vi "PSK_Mod_Receive_queue.vi"() -> ()   [LabVIEW 2014]
uses:
  <vilib>/addons/Modulation/Digital/General/MT Generate Bits (Galois, PN Order).vi
  <vilib>/addons/Modulation/Digital/Support/Common/Validators/mod_Generate Bits Validate.vi
  <vilib>/addons/Modulation/Analog/support/mod_Set Error Source.vi
  <vilib>/addons/Modulation/Digital/General/MT Generate PSK System Parameters(M).vi
  <vilib>/addons/Modulation/Digital/Support/Common/Validators/mod_Generate Filter Coefficients Validate.vi
  <vilib>/addons/Modulation/Digital/General/subVIs/mod_Generate Filter Coefficients.vi
  <vilib>/addons/Modulation/Digital/General/subVIs/mod_Generate Bits PN Sequence.vi
  <vilib>/addons/Modulation/Digital/General/MT Generate PSK Synchronization Parameters (bit array).vi
  <instrlib>/niUSRP/niUSRP Fetch Rx Data (CDB Cluster).vi
  <vilib>/addons/Modulation/niDMT.lvlib
  <vilib>/addons/Modulation/niAMT.lvlib
panel:
  out "Demod loop time":dbl
  out "USRP loop time":dbl
  out "Lost packets":u32
  in  "Header bits":i32=16
  in  "stop":bool
  out "Packets received":i32
  out "bits received":i32
  out "Aquisition time":dbl
  out "Array":i8[][](array[numeric])
  in  "Message bits":i32=128
  in  "Sync bits":i32=30
  out "sync correct?":bool
  out "output bit stream":i8[](array[numeric])
  out "Before demod&compensation":waveform(dbl)(graph)
  out "Constellation Graph":T1(graph) caption="Rx Signal Constellation"
  out "error out":errorcluster={"status"=FALSE, "code"=1074118647, "source"="niUSRP Fetch Rx Data (CDB Cluster).vi<ERR>Overflow: an internal receive buffer has filled before the data could be returned.  Consider reducing the IQ rate, increasing the Fetch rate, or increasing the number of samples per Fetch."}
  in  "USRP IP Address":refnum<k15>="192.168.10.1"
  out "Actual Rx Parameters":T2={"Rx IQ Sampling\nRate [s/sec]"=200000.0, "Rx\nFrequency [Hz]"=915000000.0, "Rx Gain [dB]"=20.0, "Rx Antenna"="RX1"} {"Rx Gain [dB]" format="%#.6p"; "Rx\nFrequency [Hz]" format="%#.6p"; "Rx IQ Sampling\nRate [s/sec]" format="%#.6p"}
  in  "Rx Parameters":T2={"Rx IQ Sampling\nRate [s/sec]"=400000.0, "Rx\nFrequency [Hz]"=5795000000.0, "Rx Gain [dB]"=0.0, "Rx Antenna"="RX1"} {"Rx Gain [dB]" format="%#.6p"; "Rx\nFrequency [Hz]" format="%#.6p"; "Rx IQ Sampling\nRate [s/sec]" format="%#.6p"}
  in  "Packets per burst":i32=20
  in  "filter parameters":T3={"Alpha"=0.5, "Filter Length"=6, "TX Filter"=enum."Root Raised Cos"} {"Alpha" format="%.2f"}
  in  "QPSK System Parameters":T4={"Samples per Symbol"=8, "symbol map"=[], "Differential PSK"=enum."disable", "PSK type"=0} {"PSK type" items=["normal", "shifted", "offset"]; "symbol map" format="%.3f"}
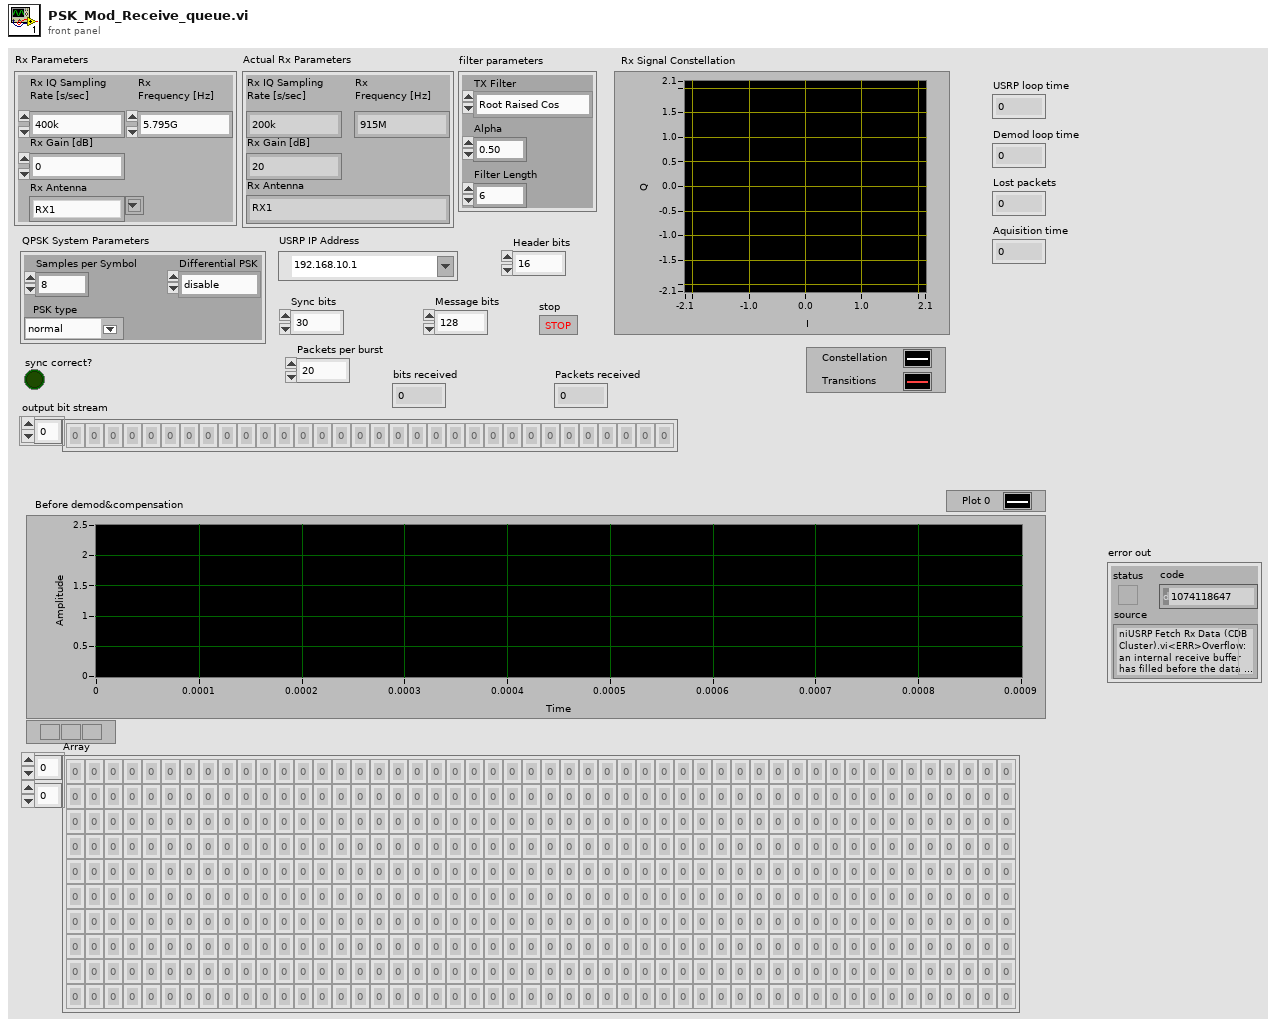
[diagram p1: front panel]
types:
  T1 = cluster{"constellation":dbl[], "oversampled data":dbl[]}[]
  T2 = cluster{"Rx IQ Sampling\nRate [s/sec]":dbl, "Rx\nFrequency [Hz]":dbl, "Rx Gain [dB]":dbl, "Rx Antenna":string}
  T3 = cluster{"Alpha":dbl, "Filter Length":i32, "TX Filter":enum16{"none", "Raised Cosine", "Root Raised Cos", "Gaussian"}}
  T4 = cluster{"Samples per Symbol":i32, "symbol map":cdb[], "Differential PSK":enum16{"disable", "enable"}, "PSK type":u16}
  T5 = enum16{"FSK", "PSK", "QAM", "MSK", "PAM", "ASK", "CPM"}
  T6 = enum16{"none", "Raised Cosine", "Root Raised Cos", "Gaussian"}
  T7 = cluster{"samples per symbol (16)":i32, "symbol map":cdb[], "differential PSK":enum16{"disable", "enable"}, "PSK type":u16}
  T8 = cluster{"expected sync location (symbols)":i32, "sync sequence":cdb[], "sync location uncertainty (symbols)":i32, "sync indent (symbols)":i32}
  T9 = typedef "niAMT.lvlib/Complex Data Waveform.ctl" = cluster{"t0":dbl, "dt":dbl, "Y":cdb[]}
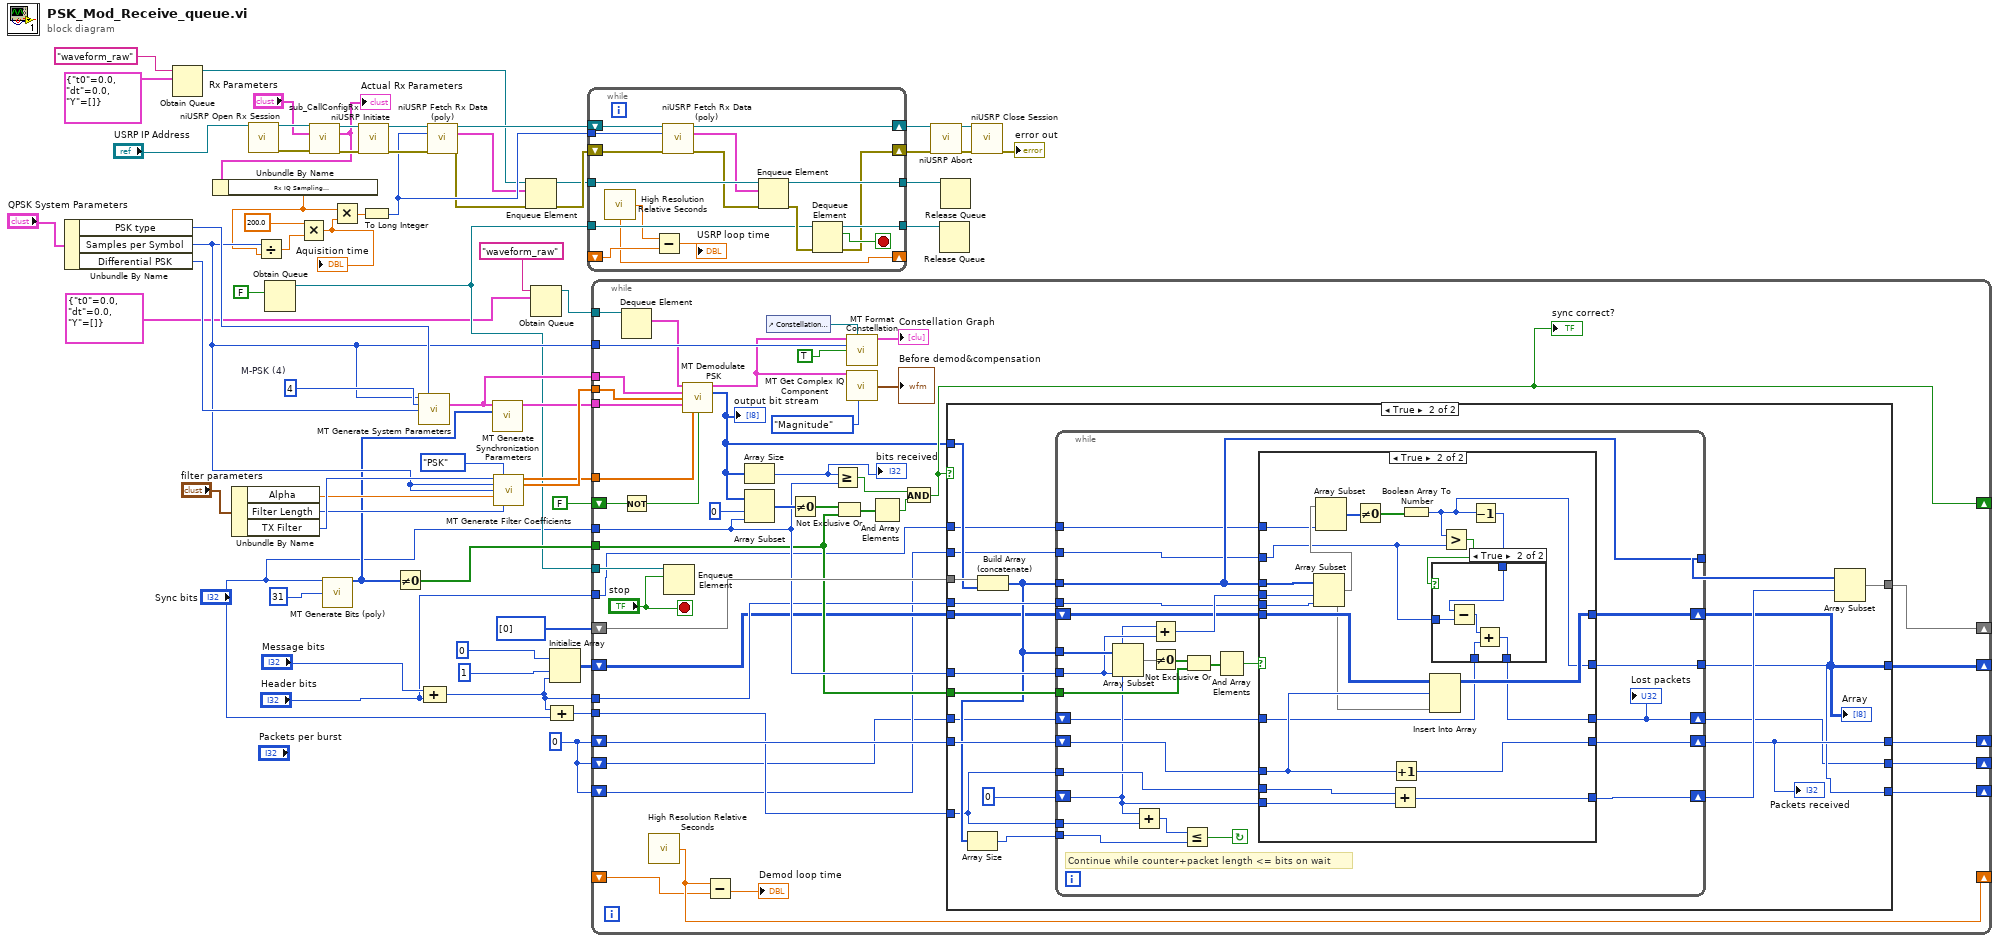
[diagram p0: block diagram]
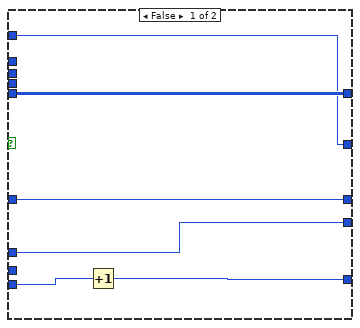
[diagram p3: hidden frame]
diagram:
  w5 = 0
  w61 = 4  # M-PSK (4)
  n1 = Unbundle By Name("QPSK System Parameters") -> ("PSK type"=w36:u16, "Samples per Symbol"=w33:i32, "Differential PSK"=w62:enum16{"disable", "enable"})
  n2 = Obtain Queue(name (unnamed)="waveform_raw", element data type=cluster{"t0":dbl, "dt":dbl, "Y":cdb[]} {"t0"=0.0, "dt"=0.0, "Y"=[]} ("data")) -> (queue out=w25:refnum<queue>)  [unwired: 3 in, 2 out]
  n3 = Unbundle By Name("filter parameters") -> ("Alpha"=w58:dbl, "Filter Length"=w59:i32, "TX Filter"=w60:T6)
  n4 = call <instrlib>:"niUSRP Open Rx Session.vi"("device names"="USRP IP Address") -> ("session handle out"=w52:refnum<k15>, "error out"=w53:errorcluster)  [unwired: 13 in]
  n5 = Obtain Queue(element data type=FALSE) -> (queue out=w12:refnum<queue>)  [unwired: 4 in, 2 out]
  n6 = call "sub_CallConfigRx.vi"("session handle"=w52, "Rx Parameters"="Rx Parameters", "error in"=w53) -> ("session handle out"=w50:refnum<k15>, "Actual Rx Parameters"=w47:T2, "error out"=w49:errorcluster)  [unwired: 10 in]
  "Actual Rx Parameters" <- w47
  n7 = Unbundle By Name(w47) -> ("Rx IQ Sampling\nRate [s/sec]"=w20:dbl)
  n8 = Divide(x=w33, y=w20) -> (x/y=w31:dbl)
  n9 = Multiply(x=200.0, y=w31) -> (x*y=w4:dbl)
  "Aquisition time" <- w4
  n10 = call-poly <vilib>:"MT Generate Bits (poly).vi"("total bits (128)"="Sync bits", "PN sequence order (9)"=31) -> ("output bit stream"=w14:i8[])  [unwired: 11 in, 2 out]
  n11 = Multiply(x=w20, y=w4) -> (x*y=w54:dbl)
  n12 = call <instrlib>:"niUSRP Initiate.vi"("session handle"=w50, "error in (no error)"=w49) -> ("session handle out"=w46:refnum<k15>, "error out"=w45:errorcluster)  [unwired: 12 in]
  n13 = To Long Integer(number=w54) -> (32bit integer=w38:i32)
  n14 = Not Equal To 0?(x=w14) -> (x != 0?=w13:bool[])
  n15 = call-poly <vilib>:"MT Generate System Parameters.vi"("samples per symbol (16)"=w33, "PSK type"=w36, "M-PSK (4)"=w61, "differential PSK"=w62) -> ("PSK system parameters"=w35:T7)  [unwired: 9 in, 2 out]
  n16 = Compound Arithmetic op=ADD("Message bits", "Header bits") -> (w7:i32)
  n17 = call-poly <instrlib>:"niUSRP Fetch Rx Data (poly).vi"("session handle"=w46, "number of samples"=w38, "error in (no error)"=w45) -> ("session handle out"=w41:refnum<k15>, "data"=w23:cluster{"t0":dbl, "dt":dbl, "Y":cdb[]}, "error out"=w22:errorcluster)  [unwired: 9 in, 1 out]
  n18 = call-poly <vilib>:"MT Generate Synchronization Parameters.vi"("PSK system parameters"=w35, "sync bits"=w14) -> ("PSK synchronization parameters"=w34:T8)  [unwired: 12 in, 1 out]
  n19 = call <vilib>:"MT Generate Filter Coefficients.vi"("pulse shaping filter (none)"=w60, "modulation type"=T5."PSK", "pulse shaping samples per symbol (16)"=w33, "matched samples per symbol (16)"=w33, "filter parameter"=w58, "filter length (symbols)"=w59) -> ("pulse shaping filter coefficients"=w30:dbl[], "matched filter coefficients"=w37:dbl[])  [unwired: 7 in, 1 out]
  n20 = Enqueue Element(queue=w25, element=w23, error in (no error)=w22) -> (queue out=w21:refnum<queue>, error out=w24:errorcluster)  [unwired: 1 in, 1 out]
  n21 = Obtain Queue(name (unnamed)="waveform_raw", element data type=cluster{"t0":dbl, "dt":dbl, "Y":cdb[]} {"t0"=0.0, "dt"=0.0, "Y"=[]} ("data")) -> (queue out=w3:refnum<queue>)  [unwired: 3 in, 2 out]
  n22 = Initialize Array(i8 0 ("element"), 1 ("dimension size"), w7) -> (w11:i8[][])
  n23 = Compound Arithmetic op=ADD(w7, "Sync bits") -> (w8:i32)
  n24 = while {
    tunnel: w38 -> [w76]
    shift-right: [w78] -> w40
    shift-left: w41 -> [w79]
    shift-right: [w69] -> w39
    shift-left: w24 -> [w77]
    tunnel: w21 -> [w75]
    tunnel: [w72] -> w17
    tunnel: [w71] -> w18
    tunnel: w12 -> [w67]
    shift-right: [w65] -> _
    shift-left: _ -> [w66]
    stop <- w70 stop-if-true
    n25 = call <vilib>:"High Resolution Relative Seconds.vi"() -> ("relative seconds"=w65:dbl)
    n26 = Subtract(x=w65, y=w66) -> (x-y=→"USRP loop time":dbl)
    n27 = call-poly <instrlib>:"niUSRP Fetch Rx Data (poly).vi"("session handle"=w79, "number of samples"=w76, "error in (no error)"=w77) -> ("session handle out"=w78:refnum<k15>, "data"=w74:cluster{"t0":dbl, "dt":dbl, "Y":cdb[]}, "error out"=w73:errorcluster)  [unwired: 9 in, 1 out]
    n28 = Enqueue Element(queue=w75, element=w74, error in (no error)=w73) -> (queue out=w72:refnum<queue>, error out=w68:errorcluster)  [unwired: 1 in, 1 out]
    n29 = Dequeue Element(queue=w67, error in (no error)=w68) -> (queue out=w71:refnum<queue>, element=w70:bool, error out=w69:errorcluster)  [unwired: 1 in, 1 out]
  }
  n30 = while {
    tunnel: w37 -> [w123]
    tunnel: w35 -> [w122]
    tunnel: w34 -> [w121]
    tunnel: w33 -> [w120]
    tunnel: w30 -> [w119]
    tunnel: w3 -> [w89]
    tunnel: "Sync bits" -> [w98]
    shift-right: [w102] -> _
    shift-left: FALSE -> [w118]
    tunnel: w12 -> [w103]
    tunnel: w13 -> [w97]
    shift-right: [w92] -> _
    shift-left: w11 -> [w94]
    shift-right: [w90] -> _
    shift-left: w5 -> [w95]
    tunnel: w8 -> [w91]
    tunnel: w7 -> [w96]
    shift-right: [w93] -> _
    shift-left: i8[] [0] ("output bit stream 2") -> [w100]
    shift-right: [w87] -> _
    shift-left: w5 -> [w88]
    tunnel: "Header bits" -> [w86]
    shift-right: [w84] -> _
    shift-left: w5 -> [w85]
    shift-right: [w83] -> _
    shift-left: _ -> [w82]
    stop <- "stop" stop-if-true
    n31 = Dequeue Element(queue=w89) -> (element=w105:cluster{"t0":dbl, "dt":dbl, "Y":cdb[]})  [unwired: 2 in, 3 out]
    n32 = Not(x=w118) -> (.not. x?=w104:bool)
    n33 = call <vilib>:"High Resolution Relative Seconds.vi"() -> ("relative seconds"=w83:dbl)
    n34 = Enqueue Element(queue=w103, element="stop") -> ()  [unwired: 2 in, 3 out]
    n35 = call <vilib>:"MT Demodulate PSK.vi"("input complex waveform"=w105, "PSK system parameters"=w122, "matched filter coefficients"=w123, "synchronization parameters"=w121, "pulse shaping filter coefficients"=w119, "reset? (T)"=w104) -> ("recovered complex waveform"=w109:T9, "output bit stream"=w101:i8[])  [unwired: 5 in, 3 out]
    "output bit stream" <- w101
    n36 = Subtract(x=w83, y=w82) -> (x-y=→"Demod loop time":dbl)
    n37 = Array Size(array=w101) -> (size(s)=w99:i32)
    "bits received" <- w99
    n38 = Array Subset(array=w101, index=0, length=w98) -> (w113:i8[])
    n39 = control-ref of="Constellation Graph"() -> (w117:refnum<vi>)
    n40 = Not Equal To 0?(x=w113) -> (x != 0?=w111:bool[])
    n41 = Greater Or Equal?(x=w99, y=w98) -> (x >= y?=w107:bool)
    n42 = Not Exclusive Or(1:w97, 2:w111) -> (0:w112:bool[])
    n43 = call <vilib>:"MT Format Constellation.vi"("waveform"=w109, "constellation reference"=w117, "samples per symbol"=w120, "autoscale"=TRUE) -> ("constellation graph"=→"Constellation Graph":T1)  [unwired: 10 in, 1 out]
    n44 = call <vilib>:"MT Get Complex IQ Component.vi"("IQ data (complex) in"=w109, "component choice"=enum16{"I", "Q", "Magnitude", "Phase"}."Magnitude") -> ("CE component"=→"Before demod&compensation":waveform(dbl))  [unwired: 11 in, 2 out]
    n45 = And Array Elements(Boolean array=w112) -> (logical AND=w106:bool)
    n46 = And(x=w107, y=w106) -> (x .and. y?=w102:bool)
    "sync correct?" <- w102
    n47 = case shown="True" w102 {
      tunnel: [w128 w136] -> w93
      tunnel: w101 -> [_ w143]
      tunnel: w100 -> [w128 w144]
      tunnel: w98 -> [_ w148]
      tunnel: w97 -> [_ w147]
      tunnel: w91 -> [_ w139]
      tunnel: w96 -> [_ w146]
      tunnel: w95 -> [w127 w145]
      tunnel: [w127 w135] -> w90
      tunnel: w94 -> [w126 w137]
      tunnel: [w126 w134] -> w92
      tunnel: w88 -> [w125 w133]
      tunnel: [w125 w132] -> w87
      tunnel: w86 -> [_ w131]
      tunnel: w85 -> [w124 w130]
      tunnel: [w124 w129] -> w84
      frame False {
      }
      frame True {
        n48 = Build Array (concatenate)(w144, w143) -> (w140:i8[])
        n49 = Array Size(array=w140) -> (size(s)=w138:i32)
        n50 = while {
          tunnel: w138 -> [w175]
          shift-right: [w174] -> w141
          shift-left: 0 ("index") -> [w158]
          tunnel: w140 -> [w171]
          tunnel: w148 -> [w166]
          tunnel: w147 -> [w168]
          tunnel: w139 -> [w173]
          tunnel: w140 -> [w159]
          tunnel: w146 -> [w164]
          tunnel: w139 -> [w162]
          tunnel: [w159] -> w142
          shift-right: [w161] -> w134
          shift-left: w137 -> [w156]
          shift-right: [w155] -> w135
          shift-left: w145 -> [w163]
          tunnel: w133 -> [w154]
          tunnel: [w153] -> w132
          tunnel: w131 -> [w152]
          shift-right: [w150] -> w129
          shift-left: w130 -> [w151]
          stop <- w167 continue-if-true
          # "Continue while counter+packet length <= bits on wait"
          n51 = Array Subset(array=w171, index=w158, length=w166) -> (w157:i8[])
          n52 = Add(x=w158, y=w173) -> (x+y=w172:i32)
          n53 = Add(x=w158, y=w166) -> (x+y=w165:i32)
          n54 = Not Equal To 0?(x=w157) -> (x != 0?=w169:bool[])
          n55 = Less Or Equal?(x=w172, y=w175) -> (x <= y?=w167:bool)
          n56 = Not Exclusive Or(1:w168, 2:w169) -> (0:w170:bool[])
          n57 = And Array Elements(Boolean array=w170) -> (logical AND=w160:bool)
          n58 = case shown="True" w160 {
            tunnel: [w180 w195] -> w174
            tunnel: w158 -> [w181 w197]
            tunnel: w159 -> [_ w192]
            tunnel: w165 -> [_ w201]
            tunnel: w164 -> [_ w200]
            tunnel: w163 -> [w179 w199]
            tunnel: [w179 w198] -> w155
            tunnel: w162 -> [_ w196]
            tunnel: w156 -> [w178 w194]
            tunnel: [w178 w193] -> w161
            tunnel: w154 -> [w177 w186]
            tunnel: [w177 w183] -> w153
            tunnel: w152 -> [_ w188]
            tunnel: w151 -> [w176 w184]
            tunnel: [w176 w182] -> w150
            frame False {
              n59 = Increment(x=w181) -> (x+1=w180:i32)
            }
            frame True {
              n60 = Array Subset(array=w192, index=w201, length=w200) -> (w191:i8[])
              n61 = Array Subset(array=w191, length=w188) -> (w189:i8[])  [unwired: 1 in]
              n62 = Not Equal To 0?(x=w189) -> (x != 0?=w190:bool[])
              n63 = Add(x=w196, y=w197) -> (x+y=w195:i32)
              n64 = Increment(x=w199) -> (x+1=w198:i32)
              n65 = Boolean Array To Number(Boolean array=w190) -> (number=w183:u32)
              n66 = Insert Into Array(array=w194, index (row)=w199, new element=w191) -> (w193:i8[][])  [unwired: 1 in]
              n67 = Greater?(x=w183, y=w186) -> (0:w187:bool)
              n68 = Decrement(x=w183) -> (x-1=w185:u32)
              n69 = case shown="True" w187 {
                tunnel: w186 -> [_ w205]
                tunnel: w185 -> [_ w206]
                tunnel: w184 -> [w202 w204]
                tunnel: [w202 w203] -> w182
                frame False {
                }
                frame True {
                  n70 = Subtract(x=w206, y=w205) -> (x-y=w207:u32)
                  n71 = Add(x=w207, y=w204) -> (x+y=w203:u32)
                }
              }
            }
          }
          "Lost packets" <- w150
        }
        "Packets received" <- w135
        "Array" <- w134
        n72 = Array Subset(array=w142, index=w141) -> (w136:i8[])  [unwired: 1 in]
      }
    }
  }
  n73 = call <instrlib>:"niUSRP Abort.vi"("session handle"=w40, "error in (no error)"=w39) -> ("session handle out"=w43:refnum<k15>, "error out"=w44:errorcluster)  [unwired: 12 in]
  n74 = Release Queue(queue=w18) -> ()  [unwired: 2 in, 3 out]
  n75 = Release Queue(queue=w17) -> ()  [unwired: 2 in, 3 out]
  n76 = call <instrlib>:"niUSRP Close Session.vi"("session handle"=w43, "error in (no error)"=w44) -> ("error out"=→"error out":errorcluster)  [unwired: 13 in]
